vi "Write LanguageFiles.vi"(8 "error in (no error)":errorcluster, 10 "LanguageFiles":T1, 11 "ContextData in":refnum<class "ContextData.lvclass">) -> (0 "error out":errorcluster, 3 "ContextData out":refnum<class "ContextData.lvclass">)   [LabVIEW 2019, in "ContextData.lvclass"]
uses:
  ContextData.lvclass
  ContextData.lvclass/ContextData.ctl
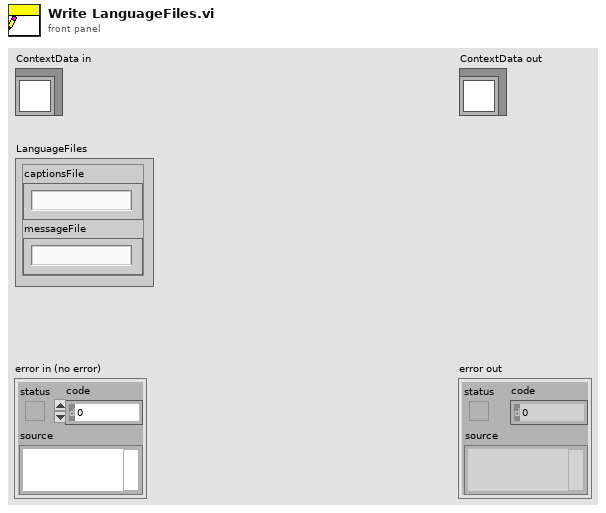
[diagram p1: front panel]
types:
  T1 = cluster{"captionsFile":string, "messageFile":string}
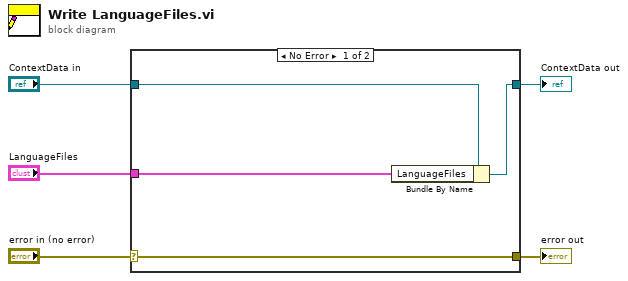
[diagram p0: block diagram]
diagram:
  n1 = case shown="No Error" "error in (no error)" {
    selector: "error in (no error)" -> [w9 w10]
    tunnel: [w9 w10] -> w4
    tunnel: [w7 w11] -> w2
    tunnel: "ContextData in" -> [w8 w11]
    tunnel: "LanguageFiles" -> [w6 _]
    frame No Error {
      n2 = Bundle By Name(cluster=w8, "LanguageFiles"=w6) -> (w7:refnum<class "ContextData.lvclass">)
    }
    frame Error {
    }
  }
  "error out" <- w4
  "ContextData out" <- w2
